vi "Read LabVIEW File Type.vi"(8 "error in (no error)":errorcluster, 11 "LabVIEW File in":refnum<class "LabVIEW File.lvclass">) -> (0 "error out":errorcluster, 2 "type":T1, 3 "LabVIEW File out":refnum<class "LabVIEW File.lvclass">)   [LabVIEW 2020, in "Save for Previous Version.lvlib" / "LabVIEW File.lvclass"]
uses:
  LabVIEW File.lvclass
  LabVIEW File.lvclass/LabVIEW File.ctl
  <vilib>/Utility/lvfile.llb/FT_FileTypes.ctl
  <vilib>/Utility/lvfile.llb/NI_FileType.lvlib
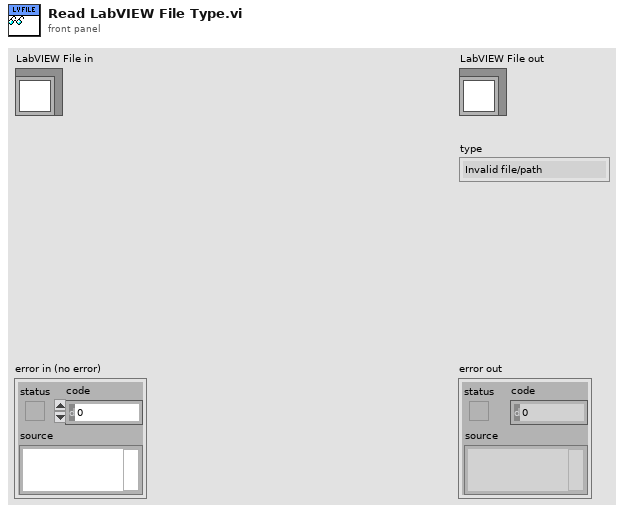
[diagram p1: front panel]
types:
  T1 = typedef "NI_FileType.lvlib/FT_FileTypes.ctl" = enum32{"Invalid file/path", "Unknown type", "Instrument", "Control", "Polymorphic VI", "Project", "Library", "LVClass", "XControl", "XNode", "CIN", "Run-time menu", "Palette menu", "LLB", "Shortcut", "Directory", "Class Private Data Control", "Statechart", "MathScript .m file", "Ladder Diagram", "LVLibp"}
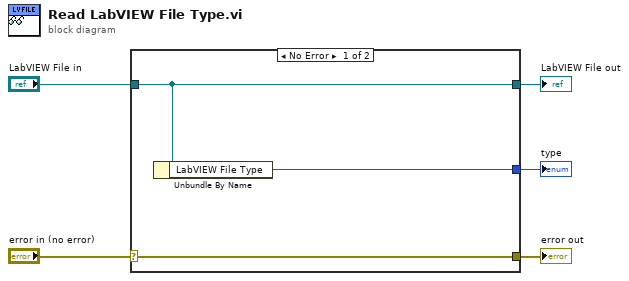
[diagram p0: block diagram]
diagram:
  n1 = case shown="No Error" "error in (no error)" {
    selector: "error in (no error)" -> [w8 w9]
    tunnel: [w8 w9] -> w4
    tunnel: [w7 w10] -> w2
    tunnel: "LabVIEW File in" -> [w7 w10]
    tunnel: [w6 _] -> w1
    frame No Error {
      n2 = Unbundle By Name(w7) -> ("LabVIEW File Type"=w6:T1)
    }
    frame Error {
    }
  }
  "error out" <- w4
  "LabVIEW File out" <- w2
  "type" <- w1
